vi "19.7-ClassicIIR-Order-Compare.vi"() -> ()   [LabVIEW 2020]
doc: "Displays the Transfer Function of the filter selected from the front panel controls. \n\nYou can select any of the 5 IIR filter design methods (Bessel, Butterworth, Chebyshev I and II, and Elliptic) and the passband type (lowpass, highpass, bandpass, and bandstop)."
uses:
  <vilib>/Analysis/3filter.llb/Filter Passband Type.ctl
  <vilib>/Analysis/NI_AALPro.lvlib
  <vilib>/Analysis/NI_AALBase.lvlib
panel:
  out "Phase":cluster{dbl, dbl, dbl[]}[](graph)
  in  "Orders":i32[](array[numeric])=[2, 3, 5, 0, 0]
  in  "LowCutoff(3dB)":dbl=250.0 format="%#.6g"
  in  "HighCutoff(3dB)":dbl=450.0 format="%#.6g"
  out "Mag":cluster{dbl, dbl, dbl[]}[](graph)
  in  "Type":T1
  in  "Stop":bool
  in  "Fs":dbl=1024.0 format="%#.6g"
  in  "Filter":T2(ring)
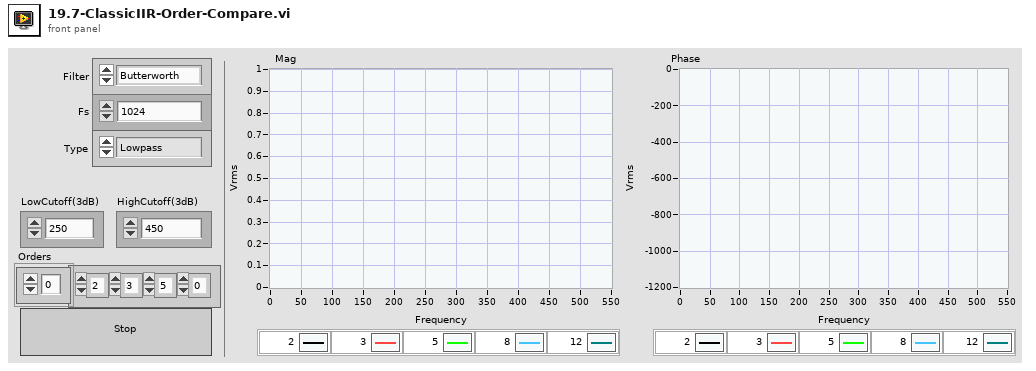
[diagram p1: front panel]
types:
  T1 = typedef "NI_AALBase.lvlib/Filter Passband Type.ctl" = enum32{"Lowpass", "Highpass", "Bandpass", "Bandstop"}
  T2 = enum16{"Butterworth", "Chebyshev", "Inverse Chebyshev", "Elliptic", "Bessel"}
  T3 = enum32{"Vrms", "Vpk", "Vrms^2", "Vpk^2", "Vrms/rtHz", "Vpk/rtHz", "Vrms^2/Hz", "Vpk^2/Hz"}
  T4 = enum16{"Power (Vrms^2)", "Amplitude (Vrms)", "Gain (amplitude ratio)"}
  T5 = cluster{"filter structure":enum32{"IIR 2nd Order", "IIR 4th Order"}, "Reverse Coefficients":dbl[], "Forward Coefficients":dbl[]}
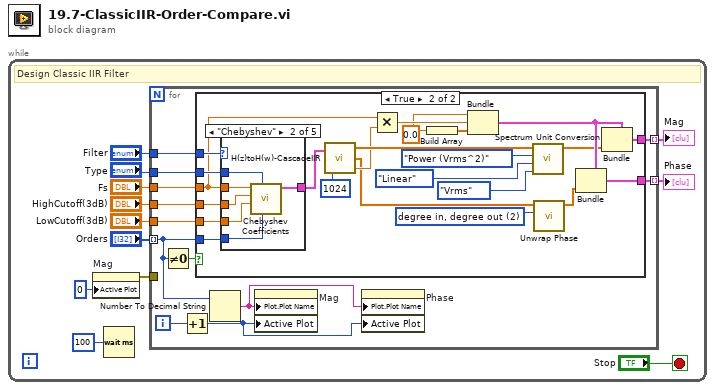
[diagram p0: block diagram]
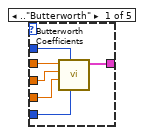
[diagram p3: hidden frame]
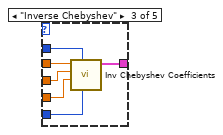
[diagram p4: hidden frame]
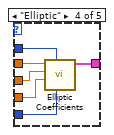
[diagram p5: hidden frame]
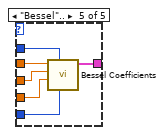
[diagram p6: hidden frame]
diagram:
  n1 = while {
    stop <- "Stop" stop-if-true
    # "Design Classic IIR Filter"
    n2 = property on="Mag" class="WFGraph (strict)"("Active Plot"=u32 0) -> (error out=w2:errorcluster)  [unwired: 2 in, 1 out]
    n3 = Wait (ms)(milliseconds to wait=u32 100) -> ()  [unwired: 1 out]
    n4 = for {
      tunnel: "Filter" -> [w24]
      tunnel: "Type" -> [w23]
      tunnel: "Fs" -> [w22]
      tunnel: [w21] -> w1 mode=indexing
      tunnel: [w20] -> w7 mode=indexing
      tunnel: "HighCutoff(3dB)" -> [w19]
      tunnel: "LowCutoff(3dB)" -> [w18]
      tunnel: "Orders" -> [w15] mode=indexing
      tunnel: w2 -> [_]
      i -> [w16]
      n5 = Not Equal To 0?(x=w15) -> (x != 0?=w17:bool)
      n6 = Increment(x=w16) -> (x+1=w13:i32)
      n7 = case shown="True" w17 {
        tunnel: w24 -> [_ w43]
        tunnel: w23 -> [_ w36]
        tunnel: w22 -> [_ w35]
        tunnel: [_ w29] -> w21
        tunnel: [_ w28] -> w20
        tunnel: w19 -> [_ w27]
        tunnel: w18 -> [_ w26]
        tunnel: w15 -> [_ w25]
        frame False {
        }
        frame True {
          w37 = 0.0
          w41 = 2 items=["radian in, radian out", "radian in, degree out", "degree in, degree out", "degree in, radian out"] ("phase unit")
          n8 = case shown="\"Chebyshev\"" w43 {
            tunnel: w36 -> [w51 w58 w65 w71 w76]
            tunnel: w35 -> [w52 w57 w63 w69 w75]
            tunnel: [w53 w59 w64 w70 w77] -> w34
            tunnel: w27 -> [w50 w56 w62 w68 w72]
            tunnel: w26 -> [w49 w55 w61 w67 w73]
            tunnel: w25 -> [w48 w54 w60 w66 w74]
            frame .."Butterworth" {
              n9 = call <vilib>:"Butterworth Coefficients.vi"("order"=w48, "filter type"=w51, "low cutoff freq: fl"=w49, "high cutoff freq: fh"=w50, "sampling freq: fs"=w52) -> ("IIR Filter Cluster"=w53:T5)  [unwired: 5 in, 1 out]
            }
            frame "Chebyshev" {
              n10 = call <vilib>:"Chebyshev Coefficients.vi"("order"=w54, "filter type"=w58, "low cutoff freq: fl"=w55, "high cutoff freq: fh"=w56, "sampling freq: fs"=w57) -> ("IIR Filter Cluster"=w59:T5)  [unwired: 5 in, 1 out]
            }
            frame "Inverse Chebyshev" {
              n11 = call <vilib>:"Inv Chebyshev Coefficients.vi"("order"=w60, "filter type"=w65, "low cutoff freq: fl"=w61, "high cutoff freq: fh"=w62, "sampling freq: fs"=w63) -> ("IIR Filter Cluster"=w64:T5)  [unwired: 5 in, 1 out]
            }
            frame "Elliptic" {
              n12 = call <vilib>:"Elliptic Coefficients.vi"("order"=w66, "filter type"=w71, "low cutoff freq: fl"=w67, "high cutoff freq: fh"=w68, "sampling freq: fs"=w69) -> ("IIR Filter Cluster"=w70:T5)  [unwired: 5 in, 1 out]
            }
            frame "Bessel".. {
              n13 = call <vilib>:"Bessel Coefficients.vi"("order"=w74, "filter type"=w76, "low cutoff freq: fl"=w73, "high cutoff freq: fh"=w72, "sampling freq: fs"=w75) -> ("IIR Filter Cluster"=w77:T5)  [unwired: 5 in, 1 out]
            }
          }
          n14 = call "H(z)toH(w)-CascadeIIR.vi"("IIR Filter Cluster"=w34, "FFT size"=1024) -> ("Mag H(w)"=w33:dbl[], "Phase H(w)"=w31:dbl[], "df"=w32:dbl)
          n15 = Multiply(x=w35, y=w32) -> (x*y=w45:dbl)
          n16 = Build Array ("array")(w37) -> (w44:dbl[])
          n17 = Bundle(w37, w45, w44) -> (w47:cluster{dbl, dbl, dbl[]})  [unwired: 1 in]
          n18 = call <vilib>:"Spectrum Unit Conversion.vi"("display unit"=T3."Vrms", "log/linear"=enum16{"Linear", "dB", "dBm"}."Linear", "spectrum type"=T4."Power (Vrms^2)", "Spectrum in"=w33) -> ("Spectrum out"=w42:dbl[])  [unwired: 6 in, 1 out]
          n19 = call <vilib>:"Unwrap Phase.vi"("phase unit"=w41, "Phase"=w31) -> ("Unwrapped Phase"=w46:dbl[])  [unwired: 8 in, 1 out]
          n20 = Bundle(cluster=w47, w46) -> (w29:cluster{dbl, dbl, dbl[]})  [unwired: 2 in]
          n21 = Bundle(cluster=w47, w42) -> (w28:cluster{dbl, dbl, dbl[]})  [unwired: 2 in]
        }
      }
      n22 = Number To Decimal String(number=w15) -> (decimal integer string=w14:string)  [unwired: 1 in]
      n23 = property on="Mag" class="WFGraph (strict)"("Plot.Plot Name"=w14, "Active Plot"=w13) -> ()  [unwired: 2 in, 2 out]
      n24 = property on="Phase" class="WFGraph (strict)"("Plot.Plot Name"=w14, "Active Plot"=w13) -> ()  [unwired: 2 in, 2 out]
    }
    "Mag" <- w7
    "Phase" <- w1
  }
